vi "Write Port Number.vi"(10 "Port Number":u16, 11 "Server in":refnum<class "Server.lvclass">) -> (3 "Server out":refnum<class "Server.lvclass">)   [LabVIEW 2016, in "Server.lvlib" / "Server.lvclass"]
uses:
  Server.lvclass
  Server.lvclass/Server.ctl
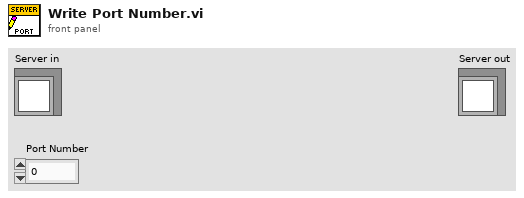
[diagram p1: front panel]
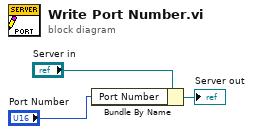
[diagram p0: block diagram]
diagram:
  n1 = Bundle By Name(cluster="Server in", "Port Number"="Port Number") -> (→"Server out":refnum<class "Server.lvclass">)
